vi "Dispatch Message.vi"(8 "error in (no error)":errorcluster, 10 "Message":refnum<class "Message.lvclass">, 11 "Manager in":refnum<class "Manager.lvclass">) -> (0 "error out":errorcluster, 3 "Manager out":refnum<class "Manager.lvclass">)   [LabVIEW 2020, in "Stream-Simple-Msg.lvlib" / "Manager.lvclass"]
uses:
  Manager.lvclass
  Message/Message.lvclass
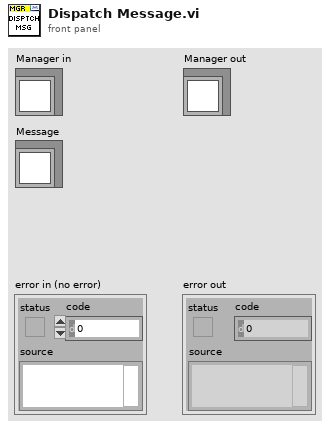
[diagram p1: front panel]
types:
  T1 = typedef "Stream-Simple-Msg.lvlib/Manager.lvclass/Callback.ctl" = cluster{"VI":refnum<vi>, "Owner":refnum<class>}
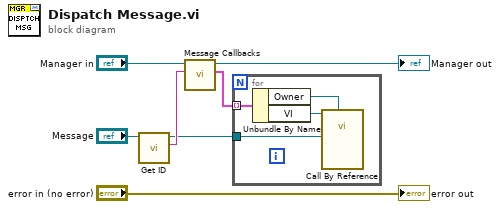
[diagram p0: block diagram]
diagram:
  n1 = call "Get ID.vi"("Message in"="Message") -> ("ID"=w5:string, "Message out"=w2:refnum<class "Message.lvclass">)  [unwired: 8 in, 1 out]
  n2 = call "Message Callbacks.vi"("Message ID"=w5, "Manager in"="Manager in") -> ("Callbacks"=w4:T1[], "Manager out"=→"Manager out":refnum<class "Manager.lvclass">)  [unwired: 7 in, 1 out]
  n3 = for {
    tunnel: w4 -> [w11] mode=indexing
    tunnel: w2 -> [w8]
    n4 = Unbundle By Name(w11) -> ("Owner"=w9:refnum<class>, "VI"=w10:refnum<vi>)
    n5 = call-by-ref "?"(reference=w10, "Owner"=w9, "Message"=w8) -> ()  [unwired: 10 in, 3 out]
  }
  "error out" <- "error in (no error)"
